vi "Exemple_Metrics_Auc.vi"() -> ()   [LabVIEW 2020]
uses:
  Objet/3 - Model selection and evaluation/3.3 - Metrics and scoring/auc/Auc.vi
panel:
  out "Score":string
  out "error out":errorcluster caption="sortie d'erreur"
  in  "error in (no error)":errorcluster caption="entrée d'erreur (pas d'erreur)"
  in  "y":string[][](array[string])=[["0,1"], ["0,4"], ["0,35"], ["0,8"]]
  in  "x":string[][](array[string])=[["1"], ["1"], ["2"], ["2"]]
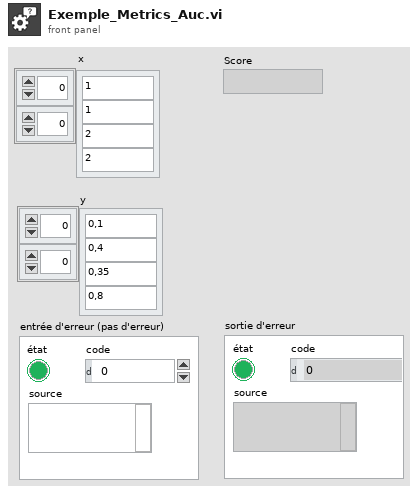
[diagram p1: front panel]
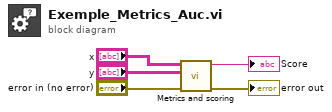
[diagram p0: block diagram]
diagram:
  n1 = call-poly "Metrics and scoring.vi"("error in (no error)"="error in (no error)", "y"="y", "x"="x") -> ("error out"=→"error out":errorcluster, "Score"=→"Score":string)  [unwired: 7 in]
